vi "SubFGV.vi"(2 "error in (no error)":errorcluster, 3 "Initial Position":dbl, 4 "Enum":T1(ring)) -> (0 "error out":errorcluster, 1 "New Position":dbl)   [LabVIEW 2019]
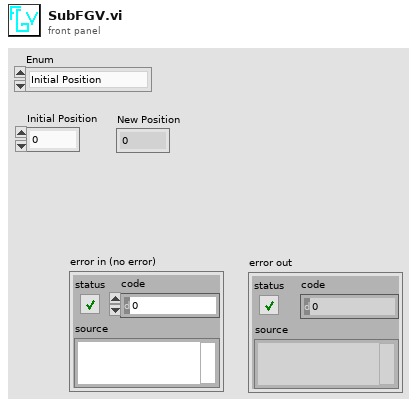
[diagram p1: front panel]
types:
  T1 = enum16{"Initial Position", "Process 1", "Process 2", "Read"}
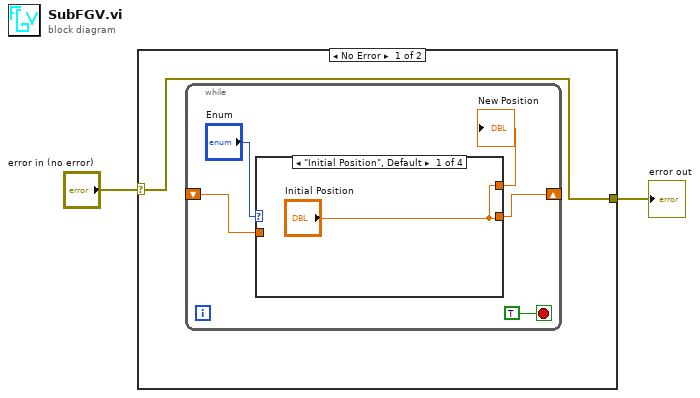
[diagram p0: block diagram]
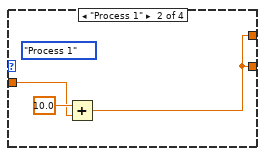
[diagram p2: hidden frame]
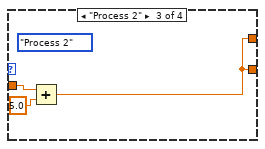
[diagram p3: hidden frame]
diagram:
  n1 = case shown="No Error" "error in (no error)" {
    selector: "error in (no error)" -> [w3 w17]
    tunnel: [w3 w17] -> w1
    frame No Error {
      n2 = while {
        shift-right: [w7] -> _
        shift-left: _ -> [w6]
        stop <- TRUE stop-if-true
        n3 = case shown="\"Initial Position\", Default" "Enum" {
          tunnel: ["Initial Position" w10 w13 w16] -> w7
          tunnel: w6 -> [_ w11 w15 w16]
          tunnel: ["Initial Position" w10 w13 w16] -> w5
          frame "Initial Position", Default {
          }
          frame "Process 1" {
            (unwired) T1."Process 1" ("Enum")
            n4 = Add(x=10.0, y=w11) -> (x+y=w10:dbl)
          }
          frame "Process 2" {
            (unwired) T1."Process 2" ("Enum")
            n5 = Add(x=w15, y=5.0) -> (x+y=w13:dbl)
          }
          frame "Read" {
          }
        }
        "New Position" <- w5
      }
    }
    frame Error {
    }
  }
  "error out" <- w1
